vi "Plot_multiplyer_and_offset.vi"(0 "Position in":dbl[](array[numeric]) format="%.2f", 1 "Increment Value":dbl=1.0 format="%.2f") -> (2 "Max Value":dbl format="%.2f", 3 "Scale":cluster{"Xo":dbl, "delta X":dbl} {"delta X" format="%.2f"; "Xo" format="%.2f"}, 4 "Position Out":dbl[](array[numeric]) format="%.2f")   [LabVIEW 2010]
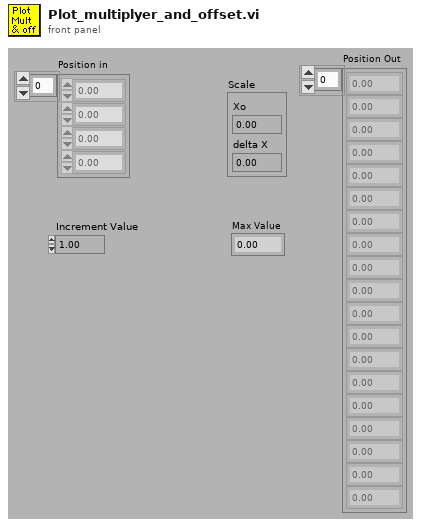
[diagram p1: front panel]
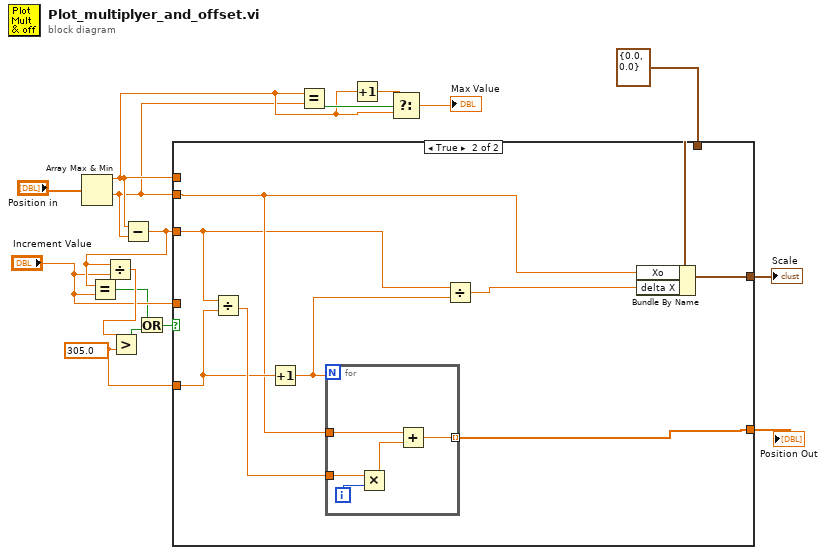
[diagram p0: block diagram]
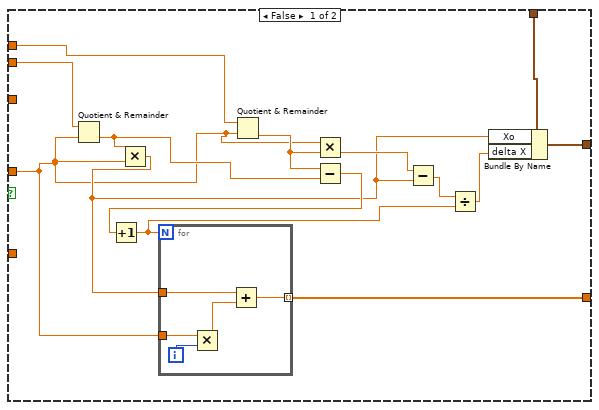
[diagram p2: hidden frame]
diagram:
  w11 = 305.0 ("y")
  n1 = Array Max & Min(array="Position in") -> (max value=w8:dbl, min value=w7:dbl)  [unwired: 2 out]
  n2 = Subtract(x=w8, y=w7) -> (x-y=w5:dbl)
  n3 = Equal?(x=w5, y="Increment Value") -> (x = y?=w2:bool)
  n4 = Divide(x=w5, y="Increment Value") -> (x/y=w12:dbl)
  n5 = Greater?(x=w12, y=w11) -> (0:w3:bool)
  n6 = Or(x=w2, y=w3) -> (x .or. y?=w1:bool)
  n7 = case shown="True" w1 {
    tunnel: [w29 w42] -> w15
    tunnel: cluster{"Xo":dbl, "delta X":dbl} {"Xo"=0.0, "delta X"=0.0} ("Write Attribute") -> [w28 w40]
    tunnel: [w27 w39] -> w13
    tunnel: w7 -> [w19 w41]
    tunnel: w8 -> [w18 _]
    tunnel: "Increment Value" -> [w17 _]
    tunnel: w5 -> [_ w37]
    tunnel: w11 -> [_ w43]
    frame False {
      n8 = Quotient & Remainder(x=w19, y=w17) -> (floor(x/y)=w30:dbl)  [unwired: 1 out]
      n9 = Multiply(x=w30, y=w17) -> (x*y=w23:dbl)
      n10 = Quotient & Remainder(x=w18, y=w17) -> (floor(x/y)=w25:dbl)  [unwired: 1 out]
      n11 = Multiply(x=w17, y=w25) -> (x*y=w24:dbl)
      n12 = Subtract(x=w25, y=w30) -> (x-y=w26:dbl)
      n13 = Increment(x=w26) -> (x+1=w21:dbl)
      n14 = for {
        N: w21 -> [_]
        tunnel: w23 -> [w35]
        tunnel: w17 -> [w33]
        tunnel: [w31] -> w29 mode=indexing
        i -> [w34]
        n15 = Multiply(x=w33, y=w34) -> (x*y=w32:dbl)
        n16 = Add(x=w35, y=w32) -> (x+y=w31:dbl)
      }
      n17 = Subtract(x=w24, y=w23) -> (x-y=w22:dbl)
      n18 = Divide(x=w22, y=w21) -> (x/y=w20:dbl)
      n19 = Bundle By Name(cluster=w28, "Xo"=w23, "delta X"=w20) -> (w27:cluster{"Xo":dbl, "delta X":dbl})
    }
    frame True {
      n20 = Divide(x=w37, y=w43) -> (x/y=w44:dbl)
      n21 = Increment(x=w43) -> (x+1=w38:dbl)
      n22 = for {
        N: w38 -> [_]
        tunnel: w41 -> [w49]
        tunnel: w44 -> [w47]
        tunnel: [w45] -> w42 mode=indexing
        i -> [w48]
        n23 = Multiply(x=w47, y=w48) -> (x*y=w46:dbl)
        n24 = Add(x=w49, y=w46) -> (x+y=w45:dbl)
      }
      n25 = Divide(x=w37, y=w38) -> (x/y=w36:dbl)
      n26 = Bundle By Name(cluster=w40, "Xo"=w41, "delta X"=w36) -> (w39:cluster{"Xo":dbl, "delta X":dbl})
    }
  }
  "Position Out" <- w15
  "Scale" <- w13
  n27 = Equal?(x=w8, y=w7) -> (x = y?=w10:bool)
  n28 = Increment(x=w8) -> (x+1=w9:dbl)
  n29 = Select(t=w9, s=w10, f=w8) -> (s? t:f=→"Max Value":dbl)
